vi "Create UDP Service.vi"(8 "error in (no error)":errorcluster, 10 "Service Details":T1, 11 "Main Display in":refnum<class "Main Display.lvclass">) -> (0 "error out":errorcluster, 3 "Main Display out":refnum<class "Main Display.lvclass">)   [LabVIEW 2016, in "Assert API Components.lvlib" / "Assert Display.lvlib" / "Main Display.lvlib" / "Main Display.lvclass"]
doc: "Configures and launches a new UDP service actor."
uses:
  Main Display.lvclass
  Service Config Display/Service Config Display/Service Details.ctl
  <vilib>/ActorFramework/Actor/Actor.lvclass
  Assert Service/Assert Service/Assert Service.lvclass
  C:/Program Files (x86)/National Instruments/LabVIEW 2016/vi.lib/ActorFramework/Actor/Actor.lvclass
  Assert Display/Assert Display.lvlib
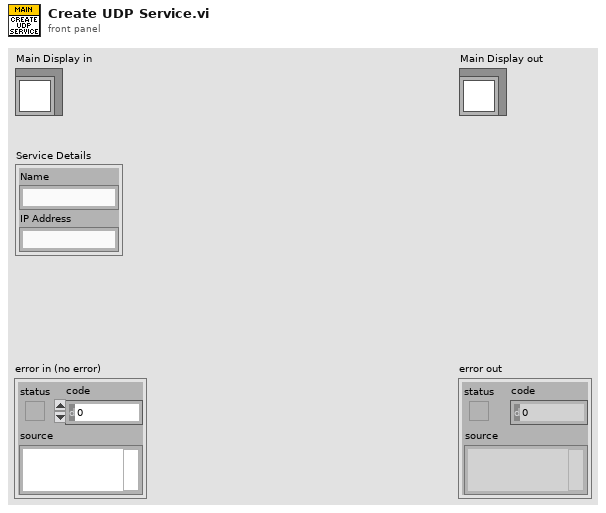
[diagram p1: front panel]
types:
  T1 = typedef "Assert API Components.lvlib/Assert Display.lvlib/Service Details.ctl" = cluster{"Name":string, "IP Address":string}
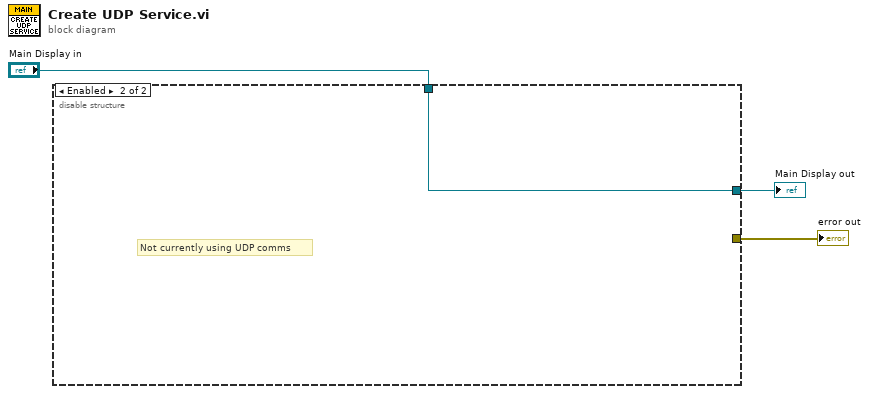
[diagram p0: block diagram]
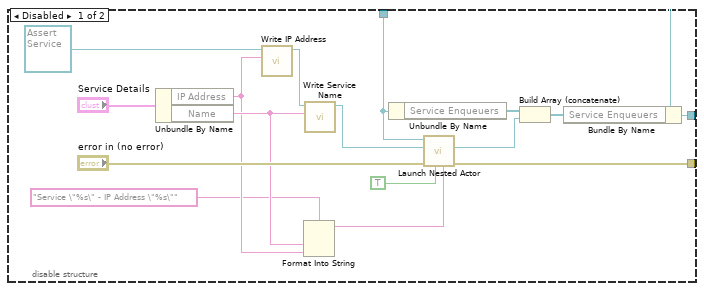
[diagram p2: hidden frame]
diagram:
  n1 = disable-structure shown="Enabled" {
    disable-tunnel: [w18 _] -> w3
    disable-tunnel: [w14 w20] -> w2
    disable-tunnel: "Main Display in" -> [w13 w20]
    frame Disabled {
      n2 = Unbundle By Name("Service Details") -> ("IP Address"=w7:string, "Name"=w8:string)
      n3 = call "Write IP Address.vi"("IP Address"=w7, "Assert Service in"=refnum<class "Assert Service.lvclass"> refnum ("Assert API Components.lvlib:Assert Service.lvlib:Assert Service.lvclass")) -> ("Assert Service out"=w16:refnum<class "Assert Service.lvclass">)  [unwired: 9 in]
      n4 = Format Into String(format string="Service \"%s\" - IP Address \"%s\"", w8, w7) -> (resulting string=w5:string)  [unwired: 2 in, 1 out]
      n5 = call "Write Service Name.vi"("Service Name"=w8, "Assert Service in"=w16) -> ("Assert Service out"=w15:refnum<class "Assert Service.lvclass">)  [unwired: 9 in]
      n6 = Unbundle By Name(w13) -> ("Service Enqueuers"=w12:refnum<class "Message Enqueuer.lvclass">[])
      n7 = call <vilib>:"Launch Nested Actor.vi"("Debug Alias"=w5, "Open Actor Core front panel? (F)"=TRUE, "error in (no error)"="error in (no error)", "Nested Actor"=w15, "Caller Actor in"=w13) -> ("error out"=w18:errorcluster, "Nested Actor's Enqueuer"=w11:refnum<class "Message Enqueuer.lvclass">)  [unwired: 4 in, 1 out]
      n8 = Build Array (concatenate)(w12, w11) -> (w10:refnum<class "Message Enqueuer.lvclass">[])
      n9 = Bundle By Name(cluster=w13, "Service Enqueuers"=w10) -> (w14:refnum<class "Main Display.lvclass">)
    }
    frame Enabled {
      # "Not currently using UDP comms"
    }
  }
  "error out" <- w3
  "Main Display out" <- w2
